vi "Camera Configuration Settings Mark2.vi"() -> ()   [LabVIEW 2019]
uses:
  <vilib>/userDefined/High Color/IMAQdx.ctl
  <vilib>/FPGAPlugInAG/myRIO-1900/niLvFpga_Open_myRIO-1900.vi
  <vilib>/rvi/interface/common/dynamic/niFpgaDynamicAddResources.vi
  <vilib>/rvi/interface/nirviOpenFPGA/nirviOpenFPGA.xnode
  Collin's Project/FPGA Bitfiles/MRmecanum_FPGATarget_FPGAMainModified_TerasRobot_LKSN2021.lvbitx
  <vilib>/vision/driver/NI_Vision_Acquisition_Software.lvlib
panel:
  out "Image":T1(plugin-control)
  in  "stop":bool
  in  "error in":errorcluster
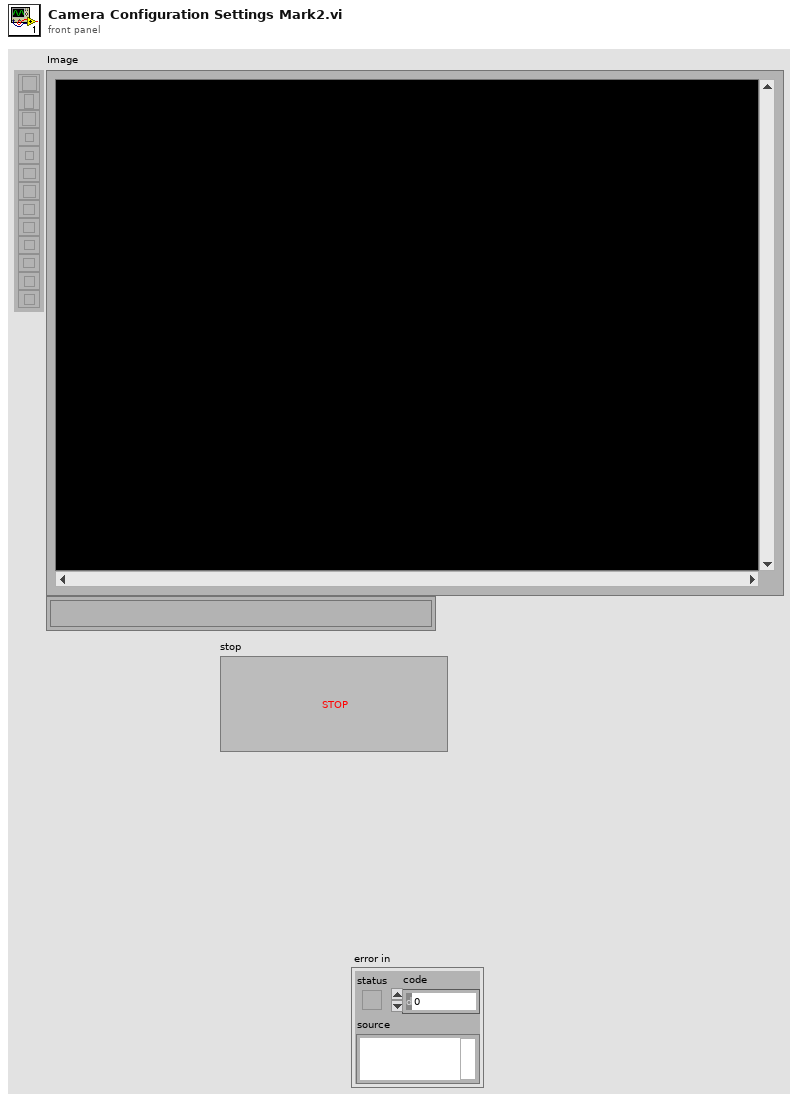
[diagram p1: front panel]
types:
  T1 = typedef "IMAQ Image.ctl" = refnum<image>
  T2 = typedef "IMAQdx.ctl" = refnum<k21>
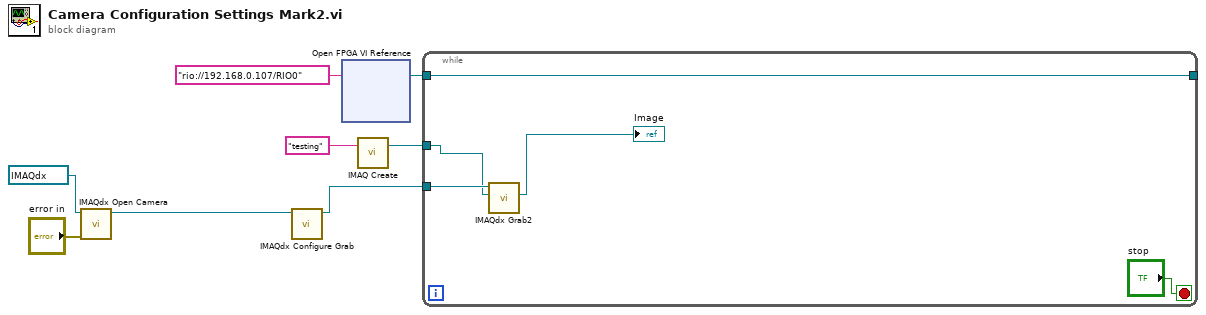
[diagram p0: block diagram]
diagram:
  n1 = call <vilib>:"IMAQdx Open Camera.vi"("error in"="error in", "Session In"=T2 "cam1") -> ("Session Out"=w2:T2)  [unwired: 8 in, 1 out]
  n2 = call <vilib>:"IMAQdx Configure Grab.vi"("Session In"=w2) -> ("Session Out"=w1:T2)  [unwired: 9 in, 1 out]
  n3 = xnode "Open FPGA VI Reference"("resource name"=tag "rio://192.168.0.107/RIO0") -> ("FPGA VI Reference Out"=w3:refnum<k20>)  [unwired: 1 in, 1 out]
  n4 = call "IMAQ Create"("Image Name"="testing") -> ("New Image"=w5:T1)  [unwired: 4 in, 1 out]
  n5 = while {
    tunnel: w5 -> [w10]
    tunnel: w3 -> [w12]
    tunnel: [w12] -> _
    tunnel: w1 -> [w11]
    stop <- "stop" stop-if-true
    n6 = call <vilib>:"IMAQdx Grab2.vi"("Image In"=w10, "Session In"=w11) -> ("Image Out"=→"Image":T1)  [unwired: 6 in, 3 out]
  }
